vi "ChSetting.vi"(9 "频率":dbl, 10 "dsc地址":string, 11 "AcquireData":waveform(dbl)[](array[waveform])) -> (1 "DexASData":T1, 2 "DevChSampData":cluster{"通道编号":string, "Data":dbl}[](array[cluster]), 3 "DevChSampleData":T2, 5 "频谱图":dbl[](graph))   [LabVIEW 2014]
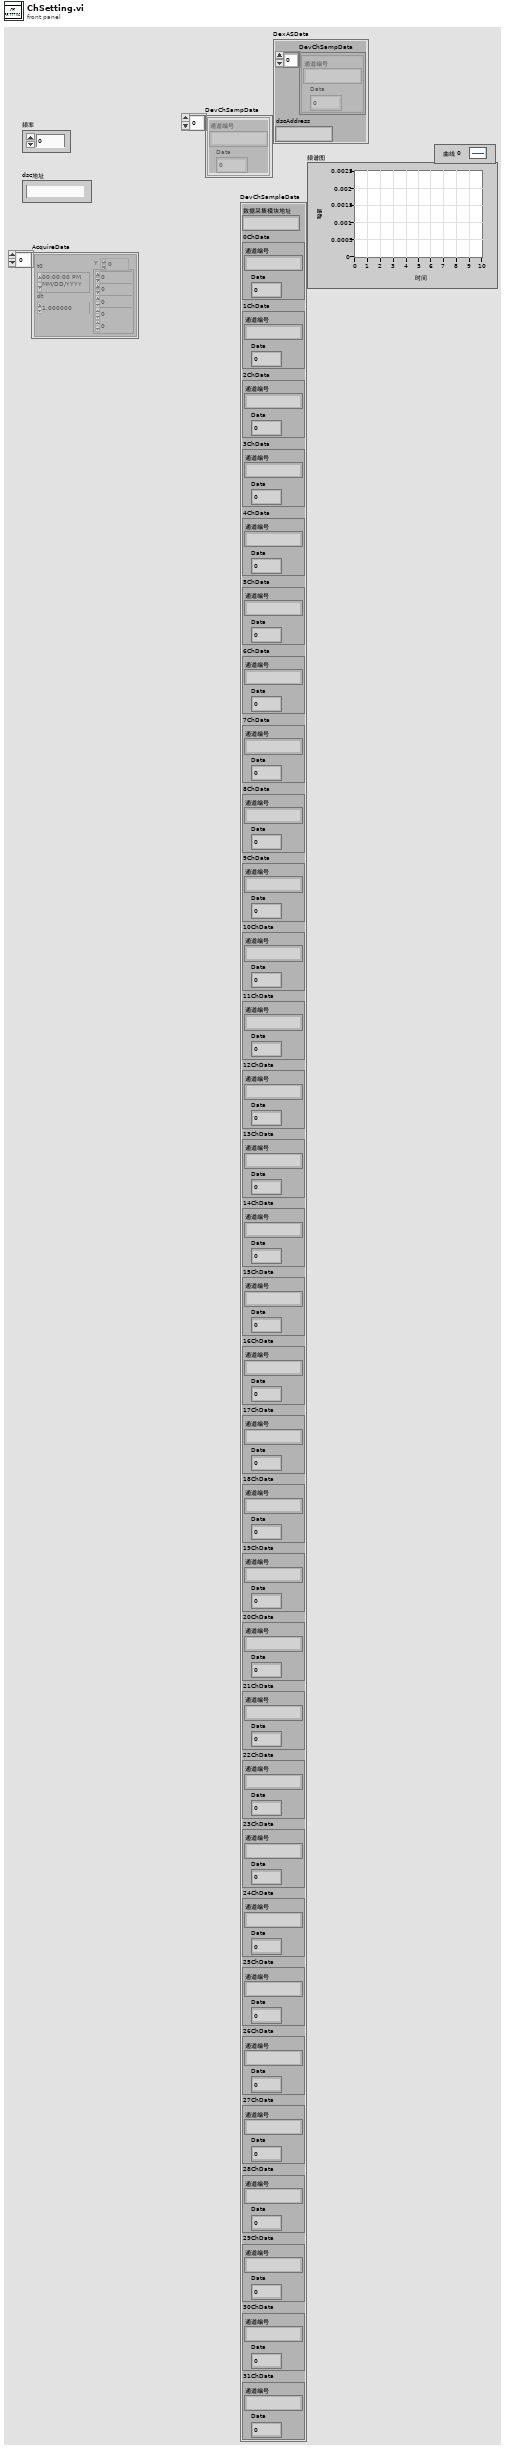
[diagram p1: front panel]
types:
  T1 = cluster{"DevChSampData":cluster{"通道编号":string, "Data":dbl}[], "dscAddress":string}
  T2 = cluster{"数据采集模块地址":string, "0ChData":cluster{"通道编号":string, "Data":dbl}, "1ChData":cluster{"通道编号":string, "Data":dbl}, "2ChData":cluster{"通道编号":string, "Data":dbl}, "3ChData":cluster{"通道编号":string, "Data":dbl}, "4ChData":cluster{"通道编号":string, "Data":dbl}, "5ChData":cluster{"通道编号":string, "Data":dbl}, "6ChData":cluster{"通道编号":string, "Data":dbl}, "7ChData":cluster{"通道编号":string, "Data":dbl}, "8ChData":cluster{"通道编号":string, "Data":dbl}, "9ChData":cluster{"通道编号":string, "Data":dbl}, "10ChData":cluster{"通道编号":string, "Data":dbl}, "11ChData":cluster{"通道编号":string, "Data":dbl}, "12ChData":cluster{"通道编号":string, "Data":dbl}, "13ChData":cluster{"通道编号":string, "Data":dbl}, "14ChData":cluster{"通道编号":string, "Data":dbl}, "15ChData":cluster{"通道编号":string, "Data":dbl}, "16ChData":cluster{"通道编号":string, "Data":dbl}, "17ChData":cluster{"通道编号":string, "Data":dbl}, "18ChData":cluster{"通道编号":string, "Data":dbl}, "19ChData":cluster{"通道编号":string, "Data":dbl}, "20ChData":cluster{"通道编号":string, "Data":dbl}, "21ChData":cluster{"通道编号":string, "Data":dbl}, "22ChData":cluster{"通道编号":string, "Data":dbl}, "23ChData":cluster{"通道编号":string, "Data":dbl}, "24ChData":cluster{"通道编号":string, "Data":dbl}, "25ChData":cluster{"通道编号":string, "Data":dbl}, "26ChData":cluster{"通道编号":string, "Data":dbl}, "27ChData":cluster{"通道编号":string, "Data":dbl}, "28ChData":cluster{"通道编号":string, "Data":dbl}, "29ChData":cluster{"通道编号":string, "Data":dbl}, "30ChData":cluster{"通道编号":string, "Data":dbl}, "31ChData":cluster{"通道编号":string, "Data":dbl}}
  T3 = cluster{"FFTch 1":dbl[], "FFTch 2":dbl[], "FFTch 3":dbl[], "FFTch 4":dbl[], "FFTch 5":dbl[], "FFTch 6":dbl[], "FFTch 7":dbl[], "FFTch 8":dbl[], "FFTch 9":dbl[], "FFTch 10":dbl[], "FFTch 11":dbl[], "FFTch 12":dbl[], "FFTch 13":dbl[], "FFTch 14":dbl[], "FFTch 15":dbl[], "FFTch 16":dbl[], "FFTch 17":dbl[], "FFTch 18":dbl[], "FFTch 19":dbl[], "FFTch 20":dbl[], "FFTch 21":dbl[], "FFTch 22":dbl[], "FFTch 23":dbl[], "FFTch 24":dbl[], "FFTch 25":dbl[], "FFTch 26":dbl[], "FFTch 27":dbl[], "FFTch 28":dbl[], "FFTch 29":dbl[], "FFTch 30":dbl[], "FFTch 31":dbl[], "FFTch 32":dbl[]}
  T4 = cluster{"value 1":dbl, "value 2":dbl, "value 3":dbl, "value 4":dbl, "value 5":dbl, "value 6":dbl, "value 7":dbl, "value 8":dbl, "value 9":dbl, "value 10":dbl, "value 11":dbl, "value 12":dbl, "value 13":dbl, "value 14":dbl, "value 15":dbl, "value 16":dbl, "value 17":dbl, "value 18":dbl, "value 19":dbl, "value 20":dbl, "value 21":dbl, "value 22":dbl, "value 23":dbl, "value 24":dbl, "value 25":dbl, "value 26":dbl, "value 27":dbl, "value 28":dbl, "value 29":dbl, "value 30":dbl, "value 31":dbl, "value 32":dbl}
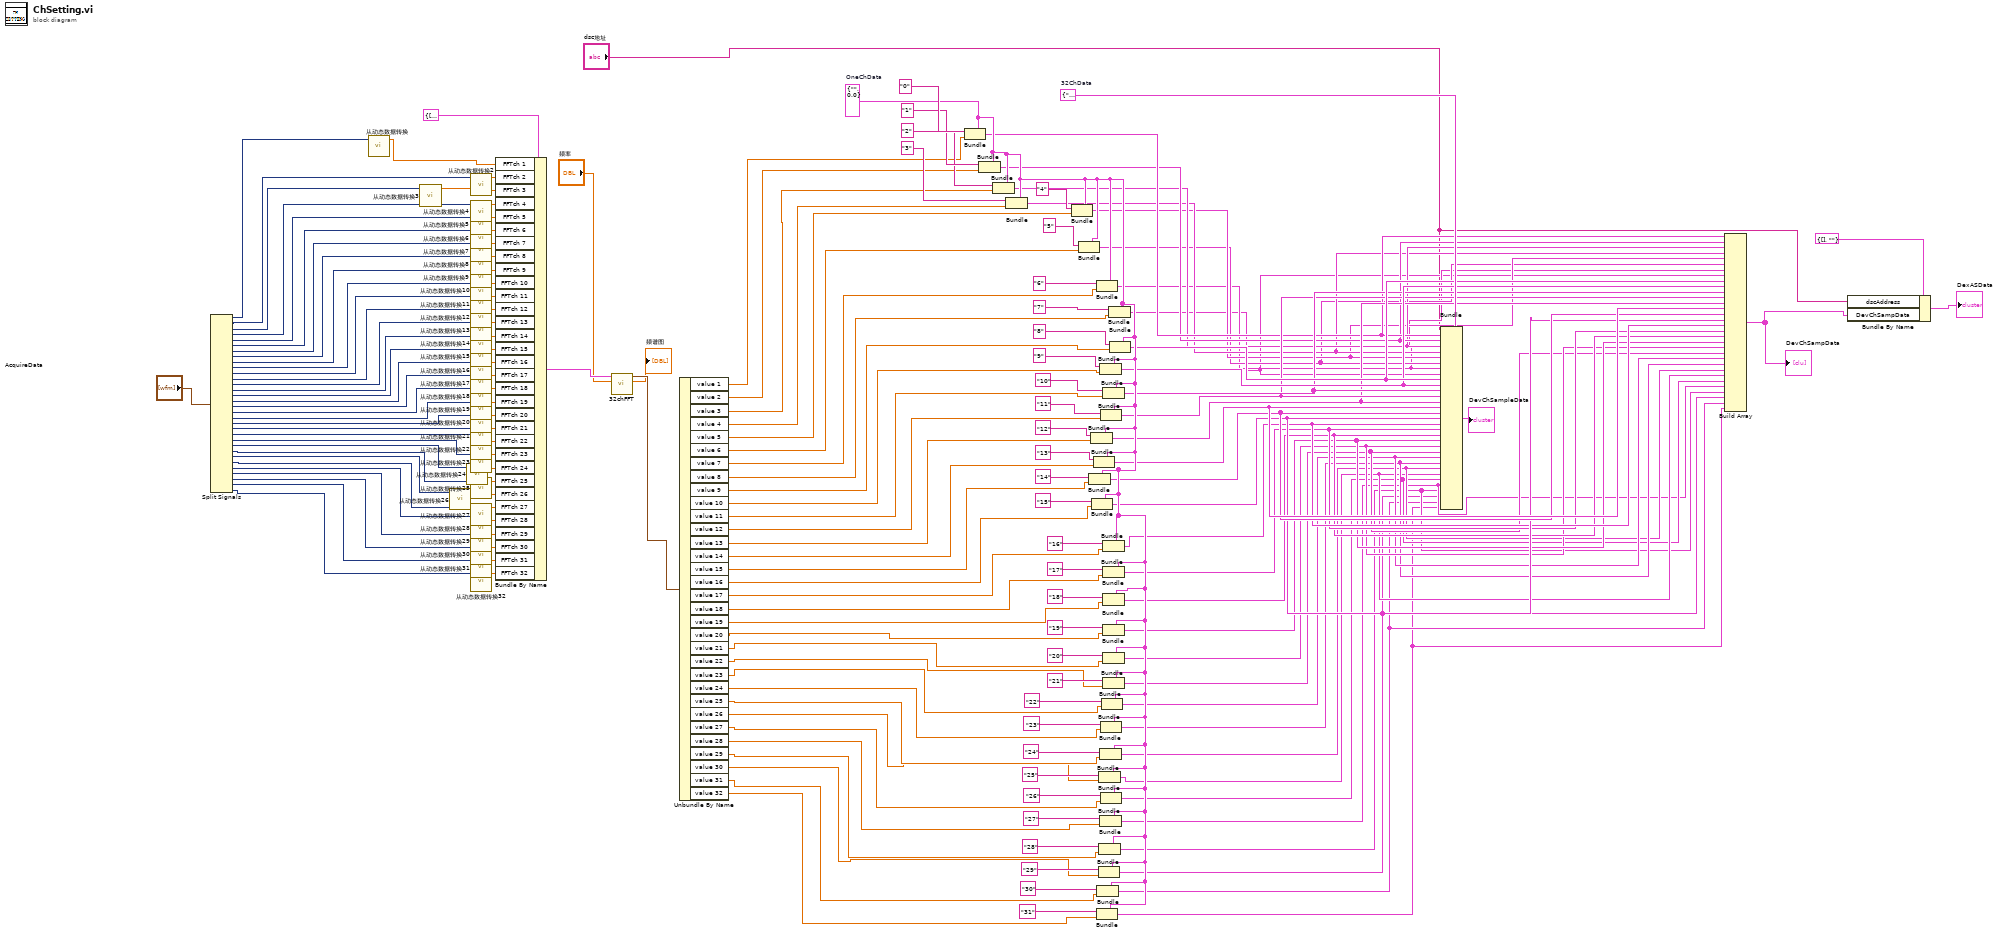
[diagram p0: block diagram]
diagram:
  w161 = T2 {"数据采集模块地址"="", "0ChData"={"通道编号"="", "Data"=0.0}, "1ChData"={"通道编号"="", "Data"=0.0}, "2ChData"={"通道编号"="", "Data"=0.0}, "3ChData"={"通道编号"="", "Data"=0.0}, "4ChData"={"通道编号"="", "Data"=0.0}, "5ChData"={"通道编号"="", "Data"=0.0}, "6ChData"={"通道编号"="", "Data"=0.0}, "7ChData"={"通道编号"="", "Data"=0.0}, "8ChData"={"通道编号"="", "Data"=0.0}, "9ChData"={"通道编号"="", "Data"=0.0}, "10ChData"={"通道编号"="", "Data"=0.0}, "11ChData"={"通道编号"="", "Data"=0.0}, "12ChData"={"通道编号"="", "Data"=0.0}, "13ChData"={"通道编号"="", "Data"=0.0}, "14ChData"={"通道编号"="", "Data"=0.0}, "15ChData"={"通道编号"="", "Data"=0.0}, "16ChData"={"通道编号"="", "Data"=0.0}, "17ChData"={"通道编号"="", "Data"=0.0}, "18ChData"={"通道编号"="", "Data"=0.0}, "19ChData"={"通道编号"="", "Data"=0.0}, "20ChData"={"通道编号"="", "Data"=0.0}, "21ChData"={"通道编号"="", "Data"=0.0}, "22ChData"={"通道编号"="", "Data"=0.0}, "23ChData"={"通道编号"="", "Data"=0.0}, "24ChData"={"通道编号"="", "Data"=0.0}, "25ChData"={"通道编号"="", "Data"=0.0}, "26ChData"={"通道编号"="", "Data"=0.0}, "27ChData"={"通道编号"="", "Data"=0.0}, "28ChData"={"通道编号"="", "Data"=0.0}, "29ChData"={"通道编号"="", "Data"=0.0}, "30ChData"={"通道编号"="", "Data"=0.0}, "31ChData"={"通道编号"="", "Data"=0.0}}  # 32ChData
  w139 = cluster{"通道编号":string, "Data":dbl} {"通道编号"="", "Data"=0.0}  # OneChData
  n1 = Split Signals("AcquireData") -> (w101:dynamicdata, w62:dynamicdata, w61:dynamicdata, w59:dynamicdata, w57:dynamicdata, w55:dynamicdata, w53:dynamicdata, w51:dynamicdata, w49:dynamicdata, w47:dynamicdata, w45:dynamicdata, w43:dynamicdata, w41:dynamicdata, w39:dynamicdata, w37:dynamicdata, w35:dynamicdata, w33:dynamicdata, w31:dynamicdata, w29:dynamicdata, w27:dynamicdata, w25:dynamicdata, w23:dynamicdata, w21:dynamicdata, w19:dynamicdata, w17:dynamicdata, w15:dynamicdata, w13:dynamicdata, w11:dynamicdata, w9:dynamicdata, w7:dynamicdata, w5:dynamicdata, w3:dynamicdata)  [unwired: 32 in]
  n2 = call "从动态数据转换"("Dynamic Data Type"=w101) -> ("Array"=w64:dbl[])  [unwired: 3 in]
  n3 = call "从动态数据转换3"("Dynamic Data Type"=w61) -> ("Array"=w60:dbl[])  [unwired: 3 in]
  n4 = call "从动态数据转换26"("Dynamic Data Type"=w15) -> ("Array"=w14:dbl[])  [unwired: 3 in]
  n5 = call "从动态数据转换24"("Dynamic Data Type"=w19) -> ("Array"=w18:dbl[])  [unwired: 3 in]
  n6 = call "从动态数据转换2"("Dynamic Data Type"=w62) -> ("Array"=w63:dbl[])  [unwired: 3 in]
  n7 = call "从动态数据转换4"("Dynamic Data Type"=w59) -> ("Array"=w58:dbl[])  [unwired: 3 in]
  n8 = call "从动态数据转换5"("Dynamic Data Type"=w57) -> ("Array"=w56:dbl[])  [unwired: 3 in]
  n9 = call "从动态数据转换6"("Dynamic Data Type"=w55) -> ("Array"=w54:dbl[])  [unwired: 3 in]
  n10 = call "从动态数据转换7"("Dynamic Data Type"=w53) -> ("Array"=w52:dbl[])  [unwired: 3 in]
  n11 = call "从动态数据转换8"("Dynamic Data Type"=w51) -> ("Array"=w50:dbl[])  [unwired: 3 in]
  n12 = call "从动态数据转换9"("Dynamic Data Type"=w49) -> ("Array"=w48:dbl[])  [unwired: 3 in]
  n13 = call "从动态数据转换10"("Dynamic Data Type"=w47) -> ("Array"=w46:dbl[])  [unwired: 3 in]
  n14 = call "从动态数据转换11"("Dynamic Data Type"=w45) -> ("Array"=w44:dbl[])  [unwired: 3 in]
  n15 = call "从动态数据转换12"("Dynamic Data Type"=w43) -> ("Array"=w42:dbl[])  [unwired: 3 in]
  n16 = call "从动态数据转换13"("Dynamic Data Type"=w41) -> ("Array"=w40:dbl[])  [unwired: 3 in]
  n17 = call "从动态数据转换14"("Dynamic Data Type"=w39) -> ("Array"=w38:dbl[])  [unwired: 3 in]
  n18 = call "从动态数据转换15"("Dynamic Data Type"=w37) -> ("Array"=w36:dbl[])  [unwired: 3 in]
  n19 = call "从动态数据转换16"("Dynamic Data Type"=w35) -> ("Array"=w34:dbl[])  [unwired: 3 in]
  n20 = call "从动态数据转换17"("Dynamic Data Type"=w33) -> ("Array"=w32:dbl[])  [unwired: 3 in]
  n21 = call "从动态数据转换18"("Dynamic Data Type"=w31) -> ("Array"=w30:dbl[])  [unwired: 3 in]
  n22 = call "从动态数据转换19"("Dynamic Data Type"=w29) -> ("Array"=w28:dbl[])  [unwired: 3 in]
  n23 = call "从动态数据转换20"("Dynamic Data Type"=w27) -> ("Array"=w26:dbl[])  [unwired: 3 in]
  n24 = call "从动态数据转换21"("Dynamic Data Type"=w25) -> ("Array"=w24:dbl[])  [unwired: 3 in]
  n25 = call "从动态数据转换22"("Dynamic Data Type"=w23) -> ("Array"=w22:dbl[])  [unwired: 3 in]
  n26 = call "从动态数据转换23"("Dynamic Data Type"=w21) -> ("Array"=w20:dbl[])  [unwired: 3 in]
  n27 = call "从动态数据转换25"("Dynamic Data Type"=w17) -> ("Array"=w16:dbl[])  [unwired: 3 in]
  n28 = call "从动态数据转换27"("Dynamic Data Type"=w13) -> ("Array"=w12:dbl[])  [unwired: 3 in]
  n29 = call "从动态数据转换28"("Dynamic Data Type"=w11) -> ("Array"=w10:dbl[])  [unwired: 3 in]
  n30 = call "从动态数据转换29"("Dynamic Data Type"=w9) -> ("Array"=w8:dbl[])  [unwired: 3 in]
  n31 = call "从动态数据转换30"("Dynamic Data Type"=w7) -> ("Array"=w6:dbl[])  [unwired: 3 in]
  n32 = call "从动态数据转换31"("Dynamic Data Type"=w5) -> ("Array"=w4:dbl[])  [unwired: 3 in]
  n33 = call "从动态数据转换32"("Dynamic Data Type"=w3) -> ("Array"=w2:dbl[])  [unwired: 3 in]
  n34 = Bundle By Name(cluster=T3 {"FFTch 1"=[], "FFTch 2"=[], "FFTch 3"=[], "FFTch 4"=[], "FFTch 5"=[], "FFTch 6"=[], "FFTch 7"=[], "FFTch 8"=[], "FFTch 9"=[], "FFTch 10"=[], "FFTch 11"=[], "FFTch 12"=[], "FFTch 13"=[], "FFTch 14"=[], "FFTch 15"=[], "FFTch 16"=[], "FFTch 17"=[], "FFTch 18"=[], "FFTch 19"=[], "FFTch 20"=[], "FFTch 21"=[], "FFTch 22"=[], "FFTch 23"=[], "FFTch 24"=[], "FFTch 25"=[], "FFTch 26"=[], "FFTch 27"=[], "FFTch 28"=[], "FFTch 29"=[], "FFTch 30"=[], "FFTch 31"=[], "FFTch 32"=[]} ("32chFFT"), "FFTch 1"=w64, "FFTch 2"=w63, "FFTch 3"=w60, "FFTch 4"=w58, "FFTch 5"=w56, "FFTch 6"=w54, "FFTch 7"=w52, "FFTch 8"=w50, "FFTch 9"=w48, "FFTch 10"=w46, "FFTch 11"=w44, "FFTch 12"=w42, "FFTch 13"=w40, "FFTch 14"=w38, "FFTch 15"=w36, "FFTch 16"=w34, "FFTch 17"=w32, "FFTch 18"=w30, "FFTch 19"=w28, "FFTch 20"=w26, "FFTch 21"=w24, "FFTch 22"=w22, "FFTch 23"=w20, "FFTch 24"=w18, "FFTch 25"=w16, "FFTch 26"=w14, "FFTch 27"=w12, "FFTch 28"=w10, "FFTch 29"=w8, "FFTch 30"=w6, "FFTch 31"=w4, "FFTch 32"=w2) -> (w99:T3)
  n35 = call "32chFFT.vi"("频率"="频率", "32chFFT"=w99) -> ("频谱图"=→"频谱图":dbl[], "32value"=w98:T4)  [unwired: 8 in]
  n36 = Unbundle By Name(w98) -> ("value 1"=w97:dbl, "value 2"=w96:dbl, "value 3"=w95:dbl, "value 4"=w94:dbl, "value 5"=w93:dbl, "value 6"=w92:dbl, "value 7"=w91:dbl, "value 8"=w90:dbl, "value 9"=w89:dbl, "value 10"=w88:dbl, "value 11"=w87:dbl, "value 12"=w86:dbl, "value 13"=w85:dbl, "value 14"=w84:dbl, "value 15"=w83:dbl, "value 16"=w82:dbl, "value 17"=w81:dbl, "value 18"=w80:dbl, "value 19"=w79:dbl, "value 20"=w78:dbl, "value 21"=w77:dbl, "value 22"=w76:dbl, "value 23"=w75:dbl, "value 24"=w74:dbl, "value 25"=w73:dbl, "value 26"=w72:dbl, "value 27"=w71:dbl, "value 28"=w70:dbl, "value 29"=w69:dbl, "value 30"=w68:dbl, "value 31"=w67:dbl, "value 32"=w66:dbl)
  n37 = Bundle(cluster=w139, "通道编号"="0", "Data"=w97) -> (w113:cluster{"通道编号":string, "Data":dbl})
  n38 = Bundle(cluster=w139, "通道编号"="1", "Data"=w96) -> (w112:cluster{"通道编号":string, "Data":dbl})
  n39 = Bundle(cluster=w139, "通道编号"="2", "Data"=w95) -> (w111:cluster{"通道编号":string, "Data":dbl})
  n40 = Bundle(cluster=w139, "通道编号"="3", "Data"=w94) -> (w110:cluster{"通道编号":string, "Data":dbl})
  n41 = Bundle(cluster=w139, "通道编号"="4", "Data"=w93) -> (w109:cluster{"通道编号":string, "Data":dbl})
  n42 = Bundle(cluster=w139, "通道编号"="5", "Data"=w92) -> (w108:cluster{"通道编号":string, "Data":dbl})
  n43 = Bundle(cluster=w139, "通道编号"="14", "Data"=w83) -> (w131:cluster{"通道编号":string, "Data":dbl})
  n44 = Bundle(cluster=w139, "通道编号"="12", "Data"=w85) -> (w133:cluster{"通道编号":string, "Data":dbl})
  n45 = Bundle(cluster=w139, "通道编号"="15", "Data"=w82) -> (w130:cluster{"通道编号":string, "Data":dbl})
  n46 = Bundle(cluster=w139, "通道编号"="13", "Data"=w84) -> (w132:cluster{"通道编号":string, "Data":dbl})
  n47 = Bundle(cluster=w139, "通道编号"="6", "Data"=w91) -> (w107:cluster{"通道编号":string, "Data":dbl})
  n48 = Bundle(cluster=w139, "通道编号"="31", "Data"=w66) -> (w114:cluster{"通道编号":string, "Data":dbl})
  n49 = Bundle(cluster=w139, "通道编号"="30", "Data"=w67) -> (w115:cluster{"通道编号":string, "Data":dbl})
  n50 = Bundle(cluster=w139, "通道编号"="29", "Data"=w68) -> (w116:cluster{"通道编号":string, "Data":dbl})
  n51 = Bundle(cluster=w139, "通道编号"="25", "Data"=w72) -> (w120:cluster{"通道编号":string, "Data":dbl})
  n52 = Bundle(cluster=w139, "通道编号"="28", "Data"=w69) -> (w117:cluster{"通道编号":string, "Data":dbl})
  n53 = Bundle(cluster=w139, "通道编号"="9", "Data"=w88) -> (w136:cluster{"通道编号":string, "Data":dbl})
  n54 = Bundle(cluster=w139, "通道编号"="24", "Data"=w73) -> (w121:cluster{"通道编号":string, "Data":dbl})
  n55 = Bundle(cluster=w139, "通道编号"="27", "Data"=w70) -> (w118:cluster{"通道编号":string, "Data":dbl})
  n56 = Bundle(cluster=w139, "通道编号"="11", "Data"=w86) -> (w134:cluster{"通道编号":string, "Data":dbl})
  n57 = Bundle(cluster=w139, "通道编号"="23", "Data"=w74) -> (w122:cluster{"通道编号":string, "Data":dbl})
  n58 = Bundle(cluster=w139, "通道编号"="26", "Data"=w71) -> (w119:cluster{"通道编号":string, "Data":dbl})
  n59 = Bundle(cluster=w139, "通道编号"="22", "Data"=w75) -> (w123:cluster{"通道编号":string, "Data":dbl})
  n60 = Bundle(cluster=w139, "通道编号"="10", "Data"=w87) -> (w135:cluster{"通道编号":string, "Data":dbl})
  n61 = Bundle(cluster=w139, "通道编号"="16", "Data"=w81) -> (w129:cluster{"通道编号":string, "Data":dbl})
  n62 = Bundle(cluster=w139, "通道编号"="17", "Data"=w80) -> (w128:cluster{"通道编号":string, "Data":dbl})
  n63 = Bundle(cluster=w139, "通道编号"="18", "Data"=w79) -> (w127:cluster{"通道编号":string, "Data":dbl})
  n64 = Bundle(cluster=w139, "通道编号"="19", "Data"=w78) -> (w126:cluster{"通道编号":string, "Data":dbl})
  n65 = Bundle(cluster=w139, "通道编号"="20", "Data"=w77) -> (w125:cluster{"通道编号":string, "Data":dbl})
  n66 = Bundle(cluster=w139, "通道编号"="21", "Data"=w76) -> (w124:cluster{"通道编号":string, "Data":dbl})
  n67 = Bundle(cluster=w139, "通道编号"="7", "Data"=w90) -> (w106:cluster{"通道编号":string, "Data":dbl})
  n68 = Bundle(cluster=w139, "通道编号"="8", "Data"=w89) -> (w137:cluster{"通道编号":string, "Data":dbl})
  n69 = Bundle(cluster=w161, "数据采集模块地址"="dsc地址", "0ChData"=w113, "1ChData"=w112, "2ChData"=w111, "3ChData"=w110, "4ChData"=w109, "5ChData"=w108, "6ChData"=w107, "7ChData"=w106, "8ChData"=w137, "9ChData"=w136, "10ChData"=w135, "11ChData"=w134, "12ChData"=w133, "13ChData"=w132, "14ChData"=w131, "15ChData"=w130, "16ChData"=w129, "17ChData"=w128, "18ChData"=w127, "19ChData"=w126, "20ChData"=w125, "21ChData"=w124, "22ChData"=w123, "23ChData"=w122, "24ChData"=w121, "25ChData"=w120, "26ChData"=w119, "27ChData"=w118, "28ChData"=w117, "29ChData"=w116, "30ChData"=w115, "31ChData"=w114) -> (→"DevChSampleData":T2)
  n70 = Build Array(w113, w112, w111, w110, w109, w108, w107, w106, w137, w136, w135, w134, w133, w132, w131, w130, w129, w128, w127, w126, w125, w124, w123, w122, w121, w120, w119, w118, w117, w116, w115, w114) -> (w103:cluster{"通道编号":string, "Data":dbl}[])
  "DevChSampData" <- w103
  n71 = Bundle By Name(cluster=T1 {"DevChSampData"=[], "dscAddress"=""} ("dscAsampledata"), "dscAddress"="dsc地址", "DevChSampData"=w103) -> (→"DexASData":T1)
